vi "setFPGAReference.vi"(10 "FPGAReference":refnum<k20>, 11 "Modbus in":refnum<class "Modbus.lvclass">) -> (3 "Modbus out":refnum<class "Modbus.lvclass">)   [LabVIEW 2015, in "Modbus.lvclass"]
uses:
  Modbus.lvclass
  Modbus.lvclass/Modbus.ctl
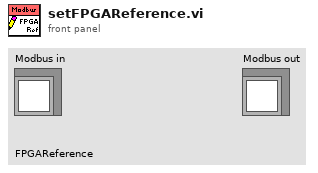
[diagram p1: front panel]
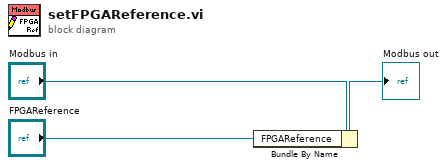
[diagram p0: block diagram]
diagram:
  n1 = Bundle By Name(cluster="Modbus in", "FPGAReference"="FPGAReference") -> (→"Modbus out":refnum<class "Modbus.lvclass">)
